vi "Device Discovery.vi"(8 "error in":errorcluster, 11 "SCADA in":refnum<class "SCADA.lvclass">) -> (0 "error out":errorcluster, 3 "SCADA out":refnum<class "SCADA.lvclass">)   [LabVIEW 2016]
uses:
  SCADA Messages/Return DeviceID Array Msg/Return DeviceID Array Msg.lvclass
  <vilib>/ActorFramework/Actor/Actor.lvclass
  SCADA Messages/Device Discovery Msg/Device Discovery Msg.lvclass
  EMS Generic Actor/EMS Generic/EMS Generic.lvclass
  SCADA.lvclass
  C:/Users/Administrator/Desktop/LabVIEW EMS/EMS Generic Actor/EMS Generic/EMS Generic.lvclass
  C:/Program Files (x86)/National Instruments/LabVIEW 2016/vi.lib/ActorFramework/Actor/Actor.lvclass
  C:/Program Files (x86)/National Instruments/LabVIEW 2016/vi.lib/ActorFramework/Message/Message.lvclass
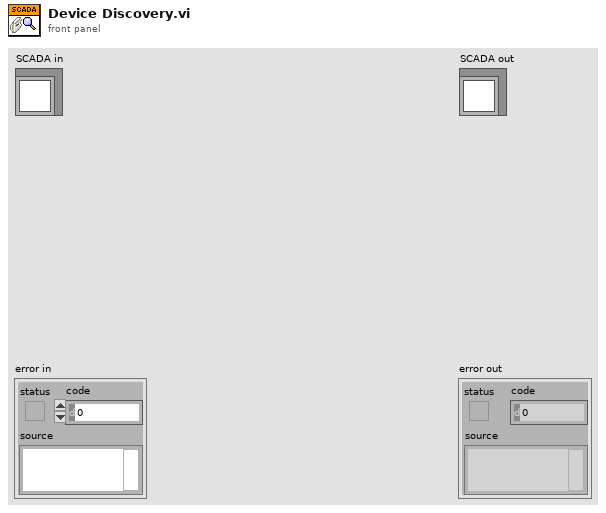
[diagram p1: front panel]
types:
  T1 = typedef "EMS Generic Actor.lvlib/EMS Generic.lvclass/Data Type DVRs.ctl" = cluster{"IED_Status":refnum<data-value>, "IED_Status_0":refnum<data-value>, "DER_Measurement":refnum<data-value>, "DER_Info":refnum<data-value>, "DER_Status":refnum<data-value>, "ES_Measurement":refnum<data-value>, "ES_Info":refnum<data-value>, "PV_Info":refnum<data-value>, "SmartRelay_Info":refnum<data-value>, "SmartRelay_Measurement":refnum<data-value>, "Meter_Info":refnum<data-value>, "Meter_Measurement":refnum<data-value>, "HVAC_Status":refnum<data-value>, "HVAC_Measurement":refnum<data-value>, "PriceData_RealTime":refnum<data-value>, "PriceData_Demand":refnum<data-value>, "PriceData_Energy":refnum<data-value>, "ForecastData_Long":refnum<data-value>, "ForecastData_Short":refnum<data-value>, "DER_Control":refnum<data-value>, "DER_SetPointF":refnum<data-value>, "DER_SetPointP":refnum<data-value>, "DER_SetPointQ":refnum<data-value>, "DER_SetPointPF":refnum<data-value>, "DER_SetPointV":refnum<data-value>, "PV_setCurtailment":refnum<data-value>, "PV_setRampRate":refnum<data-value>, "Relay_Control":refnum<data-value>, "Load_Control":refnum<data-value>, "HVAC_Control":refnum<data-value>, "Generator_Info":refnum<data-value>, "ForecastData_Long_Backup":refnum<data-value>, "PriceData_RealTime_Backup":refnum<data-value>}
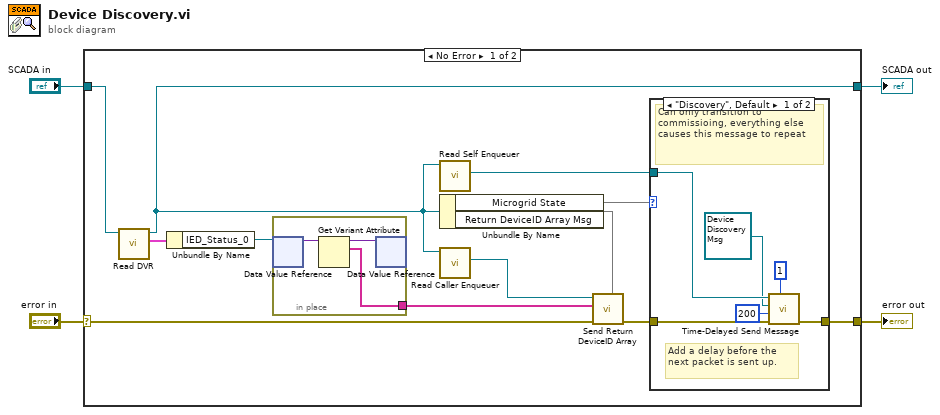
[diagram p0: block diagram]
diagram:
  n1 = case shown="No Error" "error in" {
    selector: "error in" -> [w13 w28]
    tunnel: [w9 w28] -> w3
    tunnel: [w5 w27] -> w1
    tunnel: "SCADA in" -> [w7 w27]
    frame No Error {
      n2 = call "Read DVR.vi"("EMS Generic in"=w7) -> ("DVR"=w6:T1, "EMS Generic out"=w5:refnum<class "SCADA.lvclass">)  [unwired: 9 in]
      n3 = Unbundle By Name(w6) -> ("IED_Status_0"=w16:refnum<data-value>)
      n4 = in-place {
        in-place-border: [w24] -> w8
        n5 = in-place-dvr #1(w16) -> (w26:variant)  [unwired: 1 out]
        n6 = Get Variant Attribute(Variant=w26) -> (duplicate Variant=w25:variant, names=w24:string[])  [unwired: 3 in, 2 out]
        n7 = in-place-dvr #1(w25) -> ()  [unwired: 2 out]
      }
      n8 = call <vilib>:"Read Self Enqueuer.vi"("Actor"=w5) -> ("Self Enqueuer"=w11:refnum<class "Message Enqueuer.lvclass">)  [unwired: 10 in]
      n9 = Unbundle By Name(w5) -> ("Microgrid State"=w12, "Return DeviceID Array Msg"=w14)
      n10 = call <vilib>:"Read Caller Enqueuer.vi"("Actor"=w5) -> ("Caller Enqueuer"=w15:refnum<class "Message Enqueuer.lvclass">)  [unwired: 10 in]
      n11 = call "Send Return DeviceID Array.vi"("Message Type"=w14, "error in (no error)"=w13, "DeviceID Array"=w8, "Message Enqueuer"=w15) -> ("error out"=w10:errorcluster)  [unwired: 6 in, 1 out]
      n12 = case shown="\"Discovery\", Default" w12 {
        tunnel: w11 -> [w20 _]
        tunnel: w10 -> [w22 w23]
        tunnel: [w21 w23] -> w9
        frame "Discovery", Default {
          # "Add a delay before the next packet is sent up."
          # "Can only transition to commissioing, everything else causes this message to repeat"
          n13 = call <vilib>:"Time-Delayed Send Message.vi"("# Copies (0 = infinite repeat)"=u32 1, "error in (no error)"=w22, "Milliseconds To Wait"=200, "Message"=refnum<class "Device Discovery Msg.lvclass"> refnum ("SCADA Core.lvlib:Device Discovery Msg.lvclass"), "Message Enqueuer"=w20) -> ("error out"=w21:errorcluster)  [unwired: 5 in, 1 out]
        }
        frame "Commissioning" {
          # "Once there is a state change to Commissioning, this message stops repeating."
        }
      }
    }
    frame Error {
    }
  }
  "error out" <- w3
  "SCADA out" <- w1
